vi "PathPlanner_PathConstraints_GetMaxAngularVelocity.vi"(11 "PathPlannerConstraints":T1={"MaxVelocityMps;"=0.0, "MaxAccelerationMpsSq;"=0.0, "MaxAngularVelRadPsEc;"=0.0, "MaxAngularAccRadPSecSq"=0.0, "Exists"=FALSE, "Unlimited"=FALSE, "NominalVoltageVolts"=12.0}) -> (3 "MaxAngularVelRadPsEc;":dbl)   [LabVIEW 2019, in "PathPlanner24.lvlib"]
doc: "Get max angular velocity of Path Constraints cluster\n\nInputs:\n - PathConstraint - cluster - The path constraints to query\n\nOutputs:\n - maxAngularVelocityRps - double - Max angular velocity (Rad/S)"
uses:
  PathPlanner24.lvlib
  TypeDef/PathPlannerPathConstraints.ctl
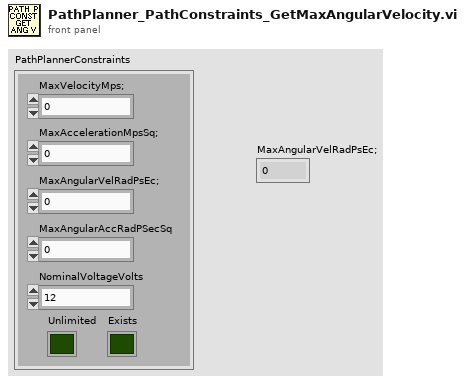
[diagram p1: front panel]
types:
  T1 = typedef "PathPlanner24.lvlib/PathPlannerPathConstraints.ctl" = cluster{"MaxVelocityMps;":dbl, "MaxAccelerationMpsSq;":dbl, "MaxAngularVelRadPsEc;":dbl, "MaxAngularAccRadPSecSq":dbl, "Exists":bool, "Unlimited":bool, "NominalVoltageVolts":dbl}
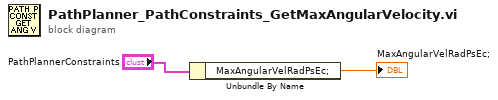
[diagram p0: block diagram]
diagram:
  n1 = Unbundle By Name("PathPlannerConstraints") -> ("MaxAngularVelRadPsEc;"=→"MaxAngularVelRadPsEc;":dbl)
